vi "Base File Path.vi"() -> (3 "Paths Out":T1)   [LabVIEW 2021]
uses:
  File Paths.ctl
panel:
  in  "Paths":T1
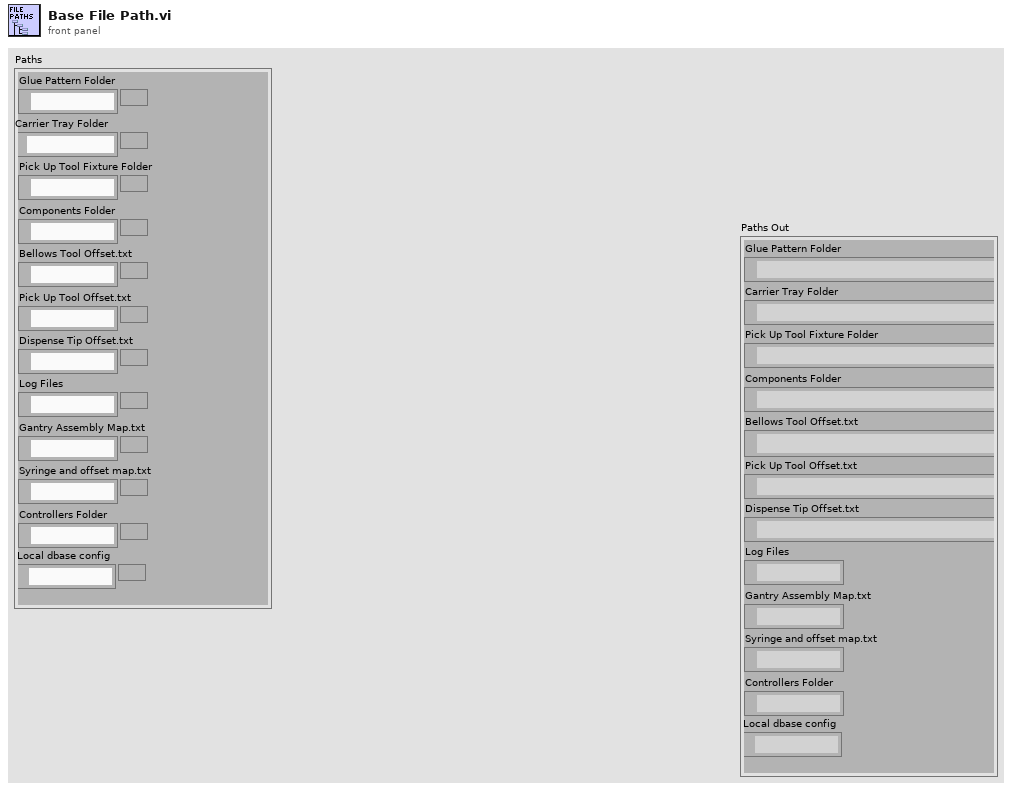
[diagram p1: front panel]
types:
  T1 = typedef "File Paths.ctl" = cluster{"Glue Pattern Folder":path, "Carrier Tray Folder":path, "Pick Up Tool Fixture Folder":path, "Components Folder":path, "Bellows Tool Offset.txt":path, "Pick Up Tool Offset.txt":path, "Dispense Tip Offset.txt":path, "Log Files":path, "Gantry Assembly Map.txt":path, "Syringe and offset map.txt":path, "Controllers Folder":path, "Local dbase config":path}
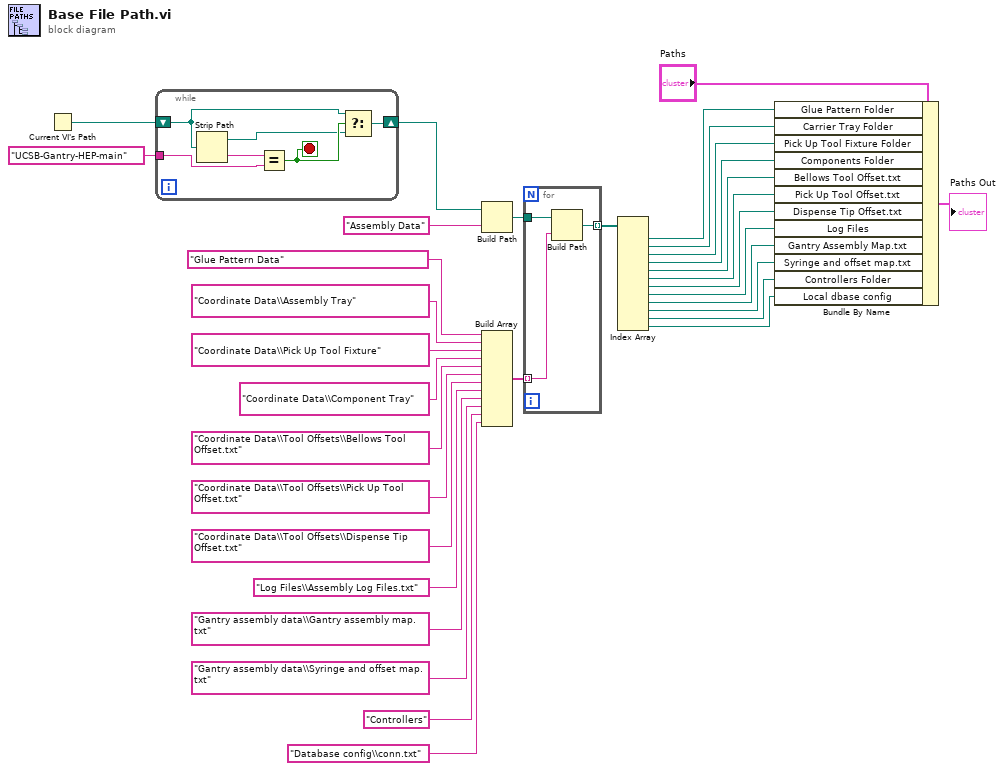
[diagram p0: block diagram]
diagram:
  n1 = Current VI's Path() -> (path=w33:path)
  n2 = while {
    shift-right: [w35] -> w29
    shift-left: w33 -> [w37]
    tunnel: "UCSB-Gantry-HEP-main" -> [w34]
    stop <- w38 stop-if-true
    n3 = Strip Path(path=w37) -> (stripped path=w36:path, name=w39:string)
    n4 = Equal?(x=w39, y=w34) -> (x = y?=w38:bool)
    n5 = Select(t=w37, s=w38, f=w36) -> (s? t:f=w35:path)
  }
  n6 = Build Path(base path=w29, name or relative path="Assembly Data") -> (appended path=w27:path)
  n7 = Build Array("Glue Pattern Data", "Coordinate Data\\Assembly Tray", "Coordinate Data\\Pick Up Tool Fixture", "Coordinate Data\\Component Tray" ("element"), "Coordinate Data\\Tool Offsets\\Bellows Tool Offset.txt", "Coordinate Data\\Tool Offsets\\Pick Up Tool Offset.txt", "Coordinate Data\\Tool Offsets\\Dispense Tip Offset.txt", "Log Files\\Assembly Log Files.txt", "Gantry assembly data\\Gantry assembly map.txt", "Gantry assembly data\\Syringe and offset map.txt", "Controllers" ("element"), "Database config\\conn.txt" ("element")) -> (w19:string[])
  n8 = for {
    tunnel: w27 -> [w42]
    tunnel: [w41] -> w31 mode=indexing
    tunnel: w19 -> [w40] mode=indexing
    n9 = Build Path(base path=w42, name or relative path=w40) -> (appended path=w41:path)
  }
  n10 = Index Array(array=w31) -> (element #1=w18:path, element #2=w17:path, element #3=w16:path, element #4=w15:path, element #5=w14:path, element #6=w13:path, element #7=w12:path, element #8=w9:path, element #9=w6:path, element #10=w5:path, element #11=w3:path, element #12=w1:path)  [unwired: 12 in]
  n11 = Bundle By Name(cluster="Paths", "Glue Pattern Folder"=w18, "Carrier Tray Folder"=w17, "Pick Up Tool Fixture Folder"=w16, "Components Folder"=w15, "Bellows Tool Offset.txt"=w14, "Pick Up Tool Offset.txt"=w13, "Dispense Tip Offset.txt"=w12, "Log Files"=w9, "Gantry Assembly Map.txt"=w6, "Syringe and offset map.txt"=w5, "Controllers Folder"=w3, "Local dbase config"=w1) -> (→"Paths Out":T1)
